vi "Read CSV File.vi"(8 "error in":errorcluster, 11 "File Path":path) -> (0 "error out":errorcluster, 3 "Data Out":dbl[][](array[numeric]) format="%0.2f")   [LabVIEW 2021]
uses:
  <vilib>/Utility/file.llb/Read Delimited Spreadsheet (DBL).vi
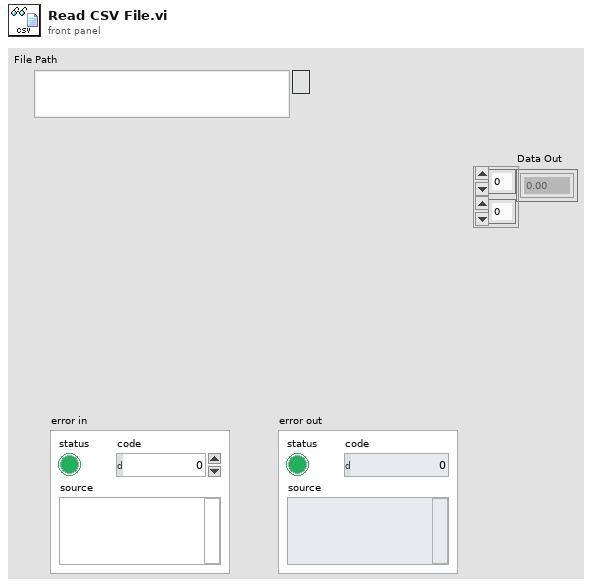
[diagram p1: front panel]
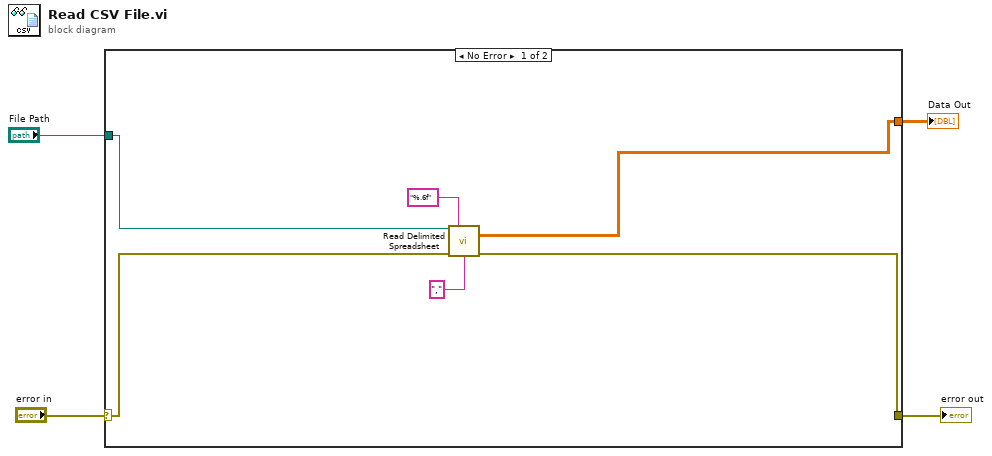
[diagram p0: block diagram]
diagram:
  n1 = case shown="No Error" "error in" {
    selector: "error in" -> [w10 w11]
    tunnel: "File Path" -> [w9 _]
    tunnel: [w7 w11] -> w2
    tunnel: [w5 _] -> w1
    frame No Error {
      n2 = call-poly <vilib>:"Read Delimited Spreadsheet.vi"("file path (dialog if empty)"=w9, "format (%.3f)"="%.6f", "error in (no error)"=w10, "delimiter (\\t)"="," ("delimiter (\\t)")) -> ("all rows"=w5:dbl[][], "error out"=w7:errorcluster)  [unwired: 6 in, 4 out]
    }
    frame Error {
    }
  }
  "error out" <- w2
  "Data Out" <- w1
